vi "Main.vi"() -> ()   [LabVIEW 2017]
uses:
  Tank Class/Tank.lvclass
  Sensor Class/Sensor.lvclass
  Pump Class/Pump.lvclass
  Pump Class/Pump.lvclass/Pump.ctl
  Sensor Class/Sensor.lvclass/Sensor.ctl
  Tank Class/Tank.lvclass/Tank.ctl
panel:
  out "Level 2":bool
  out "Level 1":bool
  out "Pump":bool
  in  "stop":bool
  out "Tank":dbl(slide) scale=0.0..100.0
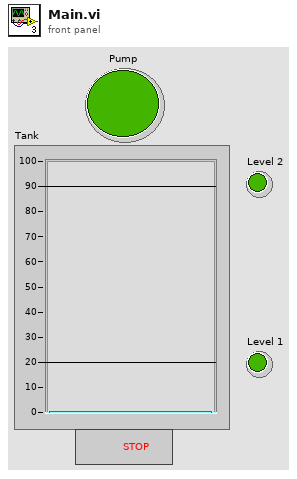
[diagram p1: front panel]
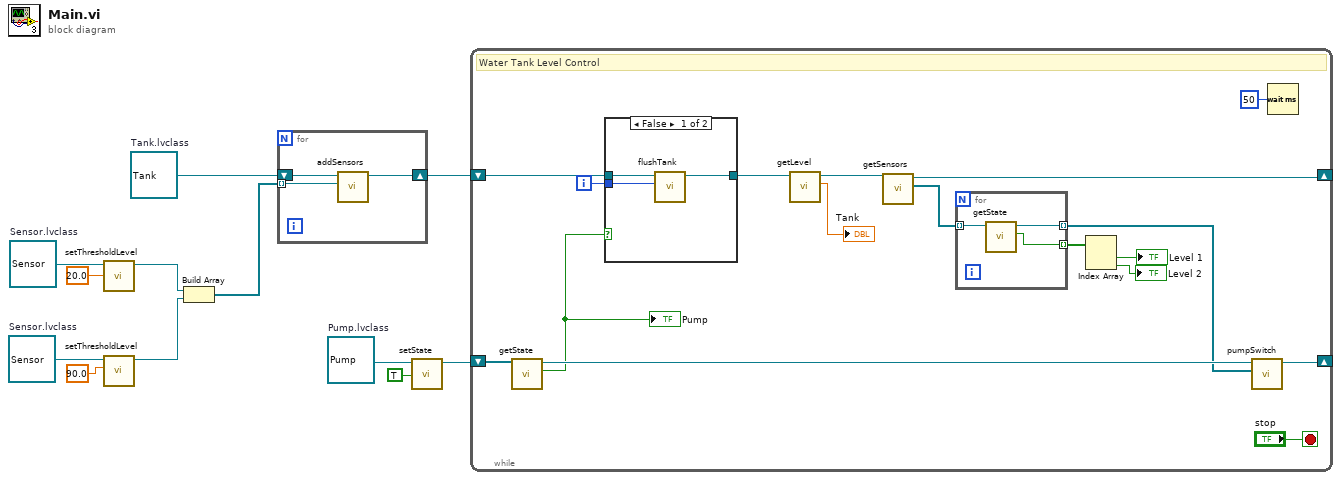
[diagram p0: block diagram]
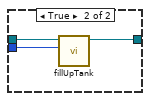
[diagram p2: hidden frame]
diagram:
  w3 = refnum<class "Pump.lvclass"> refnum  # Pump.lvclass
  w11 = refnum<class "Sensor.lvclass"> refnum  # Sensor.lvclass
  w10 = refnum<class "Sensor.lvclass"> refnum  # Sensor.lvclass
  w12 = refnum<class "Tank.lvclass"> refnum  # Tank.lvclass
  n1 = call "setThresholdLevel.vi"("Threshold Level"=20.0, "Sensor in"=w10) -> ("Sensor out"=w8:refnum<class "Sensor.lvclass">)  [unwired: 8 in, 1 out]
  n2 = call "setThresholdLevel.vi"("Threshold Level"=90.0, "Sensor in"=w11) -> ("Sensor out"=w7:refnum<class "Sensor.lvclass">)  [unwired: 8 in, 1 out]
  n3 = Build Array(w8, w7) -> (w4:refnum<class "Sensor.lvclass">[])
  n4 = for {
    shift-right: [w14] -> w9
    shift-left: w12 -> [w15]
    tunnel: w4 -> [w13] mode=indexing
    n5 = call "addSensors.vi"("Sensor.lvclass"=w13, "Tank in"=w15) -> ("Tank out"=w14:refnum<class "Tank.lvclass">)  [unwired: 8 in, 1 out]
  }
  n6 = call "setState.vi"("state"=TRUE, "Pump in"=w3) -> ("Pump out"=w2:refnum<class "Pump.lvclass">)  [unwired: 8 in, 1 out]
  n7 = while {
    shift-right: [w29] -> _
    shift-left: w2 -> [w30]
    shift-right: [w20] -> _
    shift-left: w9 -> [w27]
    i -> [w18]
    stop <- "stop" stop-if-true
    # "Water Tank Level Control"
    n8 = call "getState.vi"("Pump in"=w30) -> ("state"=w19:bool, "Pump out"=w28:refnum<class "Pump.lvclass">)  [unwired: 8 in, 1 out]
    "Pump" <- w19
    n9 = case shown="False" w19 {
      tunnel: [w34 w38] -> w32
      tunnel: w27 -> [w35 w37]
      tunnel: w18 -> [w33 w36]
      frame False {
        n10 = call "flushTank.vi"("Index"=w33, "Tank in"=w35) -> ("Tank out"=w34:refnum<class "Tank.lvclass">)  [unwired: 8 in, 1 out]
      }
      frame True {
        n11 = call "fillUpTank.vi"("Index"=w36, "Tank in"=w37) -> ("Tank out"=w38:refnum<class "Tank.lvclass">)  [unwired: 8 in, 1 out]
      }
    }
    n12 = call "getLevel.vi"("Tank in"=w32) -> ("Level"=→"Tank":dbl, "Tank out"=w17:refnum<class "Tank.lvclass">)  [unwired: 8 in, 1 out]
    n13 = call "getSensors.vi"("Tank in"=w17) -> ("Sensors"=w31:refnum<class "Sensor.lvclass">[], "Tank out"=w20:refnum<class "Tank.lvclass">)  [unwired: 8 in, 1 out]
    n14 = for {
      tunnel: w31 -> [w41] mode=indexing
      tunnel: [w40] -> w25 mode=indexing
      tunnel: [w39] -> w24 mode=indexing
      n15 = call "getState.vi"("Sensor in"=w41) -> ("State"=w39:bool, "Sensor out"=w40:refnum<class "Sensor.lvclass">)  [unwired: 8 in, 1 out]
    }
    n16 = Index Array(array=w24) -> (element #1=→"Level 1":bool, element #2=→"Level 2":bool)  [unwired: 2 in]
    n17 = call "pumpSwitch.vi"("Sensors"=w25, "Pump in"=w28) -> ("Pump out"=w29:refnum<class "Pump.lvclass">)  [unwired: 8 in, 1 out]
    n18 = Wait (ms)(milliseconds to wait=u32 50) -> ()  [unwired: 1 out]
  }
